vi "CLD 5 Parse Config Data File.vi"(8 "error in (no error)":errorcluster, 10 "Array In":T1[][](array[typedef])=[[{"Numeric"=1.25, "Boolean"=FALSE, "String"="One"}, {"Numeric"=1.35, "Boolean"=TRUE, "String"="Two"}, {"Numeric"=1.5, "Boolean"=FALSE, "String"="Three"}, {"Numeric"=1.0, "Boolean"=TRUE, "String"="Four"}], [{"Numeric"=2.0, "Boolean"=TRUE, "String"="Five"}, {"Numeric"=0.75, "Boolean"=FALSE, "String"="Six"}, {"Numeric"=0.9, "Boolean"=TRUE, "String"="Seven"}, {"Numeric"=0.75, "Boolean"=FALSE, "String"="Eight"}]], 11 "Get/Set":enum16{"Get", "Set"}(ring)) -> (0 "error out":errorcluster, 3 "Array Out":T1[][](array[typedef]))   [LabVIEW 2025]
doc: "CLD 5 exercise"
uses:
  CLD 5 Data Cluster.ctl
  <vilib>/Utility/config.llb/Read Key (Double).vi
  <vilib>/Utility/config.llb/Read Key (String).vi
  <vilib>/Utility/config.llb/Read Key (Boolean).vi
  <vilib>/Utility/config.llb/Read Key (I32).vi
  <vilib>/Utility/config.llb/Write Key (I32).vi
  <vilib>/Utility/config.llb/Write Key (String).vi
  <vilib>/Utility/config.llb/Write Key (Boolean).vi
  <vilib>/Utility/config.llb/Write Key (Double).vi
  <vilib>/Utility/config.llb/NI_LVConfig.lvlib
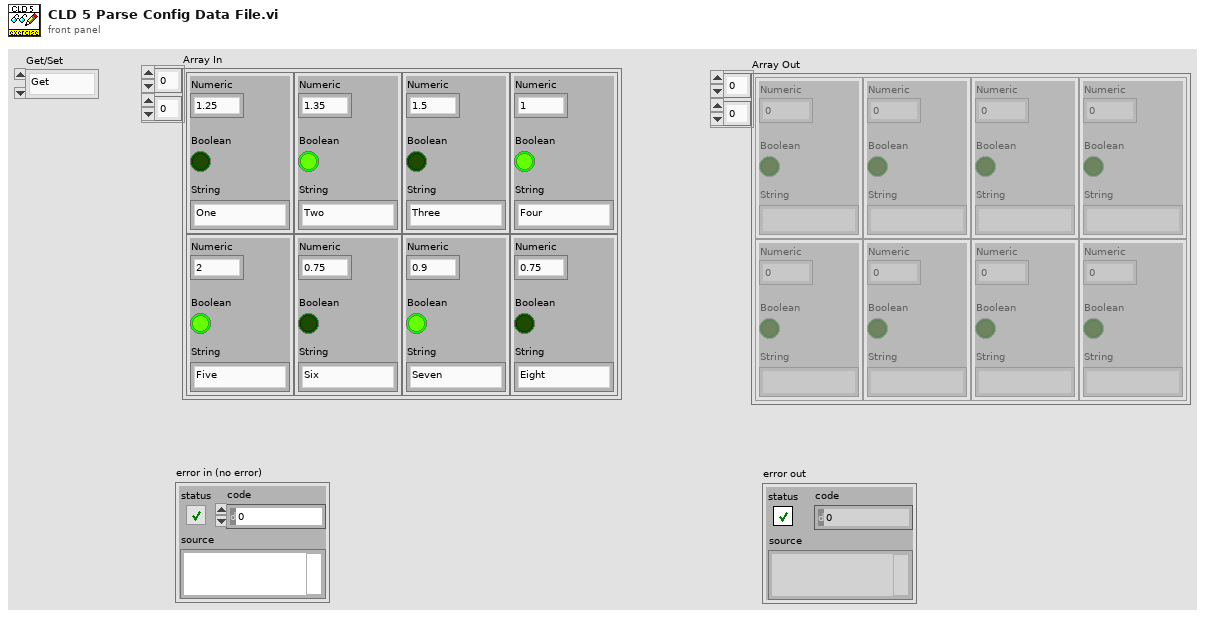
[diagram p1: front panel]
types:
  T1 = typedef "CLD 5 Data Cluster.ctl" = cluster{"Numeric":dbl, "Boolean":bool, "String":string}
  T2 = typedef "NI_LVConfig.lvlib/Config Data RefNum.ctl" = refnum<k1>
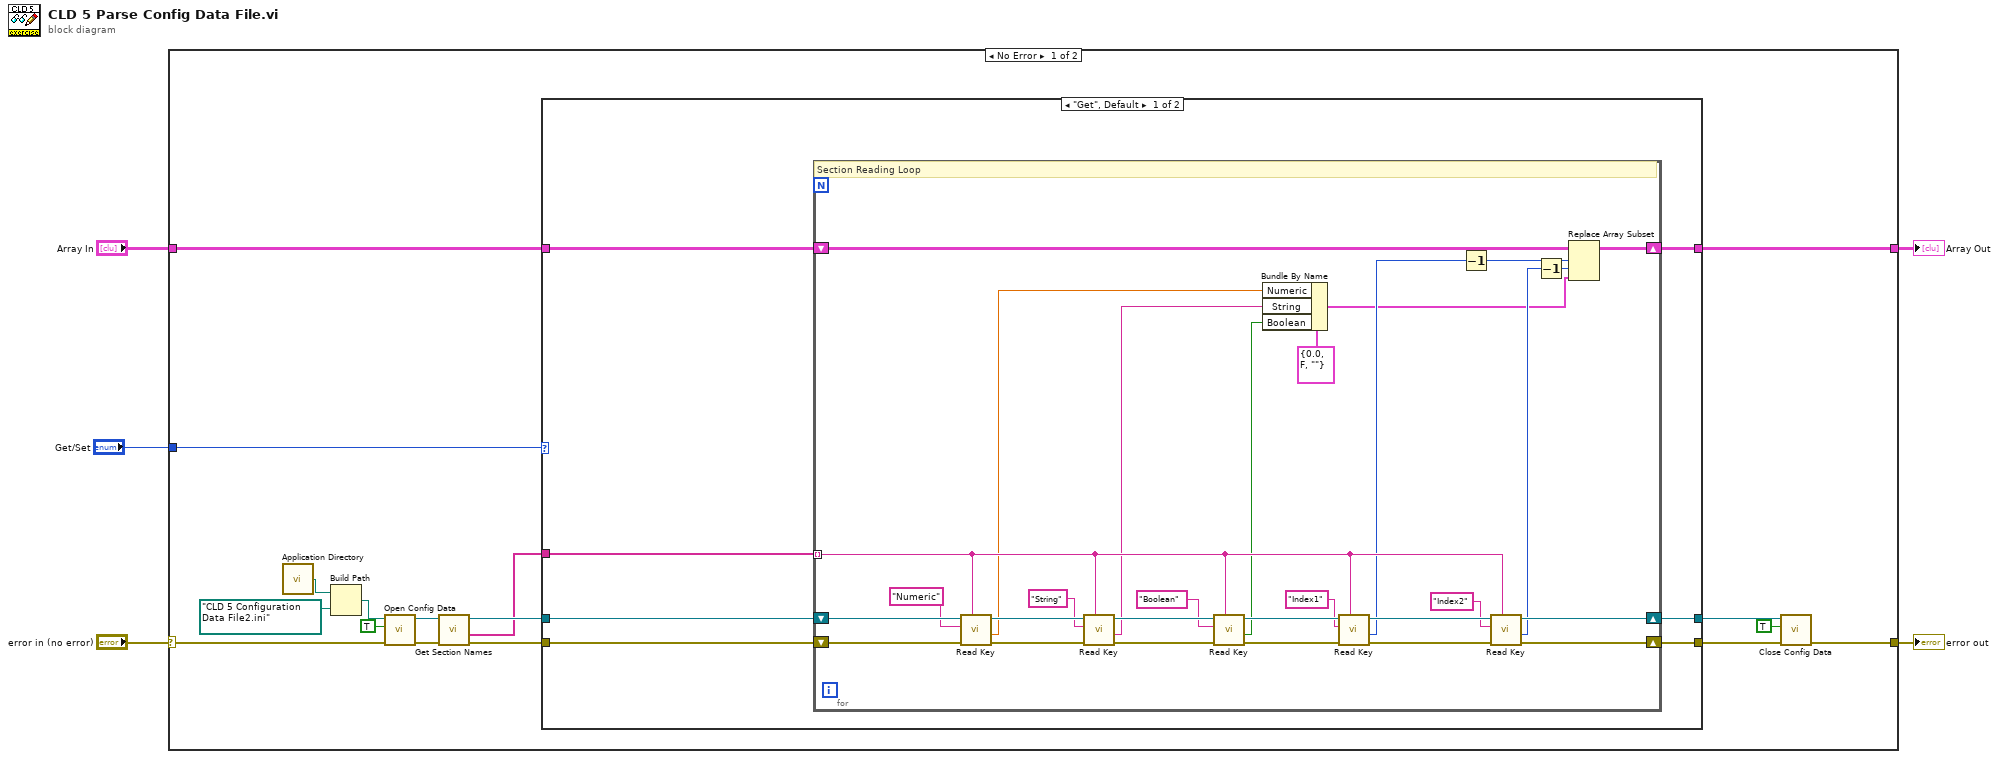
[diagram p0: block diagram]
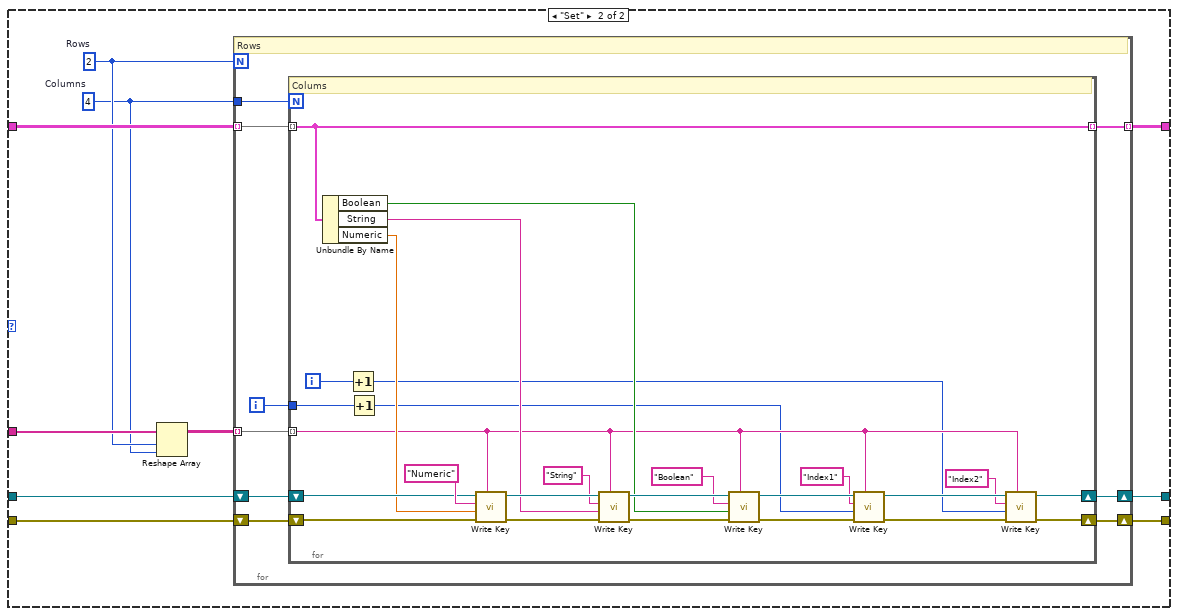
[diagram p2: hidden frame]
diagram:
  n1 = case shown="No Error" "error in (no error)" {
    selector: "error in (no error)" -> [w22 w105]
    tunnel: [w16 w105] -> w4
    tunnel: "Array In" -> [w20 w104]
    tunnel: [w19 w104] -> w2
    tunnel: "Get/Set" -> [w18 _]
    frame No Error {
      n2 = call <vilib>:"Application Directory.vi"() -> ("Application Directory"=w13:path)
      n3 = Build Path(base path=w13, name or relative path=path "CLD 5 Configuration Data File2.ini") -> (appended path=w14:path)
      n4 = call <vilib>:"Open Config Data.vi"("error in (no error)"=w22, "create file if necessary (T)"=TRUE, "configuration file path"=w14) -> ("error out"=w17:errorcluster, "refnum"=w9:T2)  [unwired: 6 in, 1 out]
      n5 = call <vilib>:"Get Section Names.vi"("error in (no error)"=w17, "refnum"=w9) -> ("error out"=w10:errorcluster, "section names"=w7:string[], "refnum out"=w8:T2)  [unwired: 7 in]
      n6 = case shown="\"Get\", Default" w18 {
        tunnel: w10 -> [w28 w68]
        tunnel: [w25 w65] -> w21
        tunnel: w20 -> [w29 w67]
        tunnel: [w26 w66] -> w19
        tunnel: w8 -> [w24 w64]
        tunnel: [w27 w63] -> w15
        tunnel: w7 -> [w23 w62]
        frame "Get", Default {
          n7 = for {
            shift-right: [w53] -> w25
            shift-left: w28 -> [w57]
            shift-right: [w55] -> w27
            shift-left: w24 -> [w56]
            tunnel: w23 -> [w44] mode=indexing
            shift-right: [w54] -> w26
            shift-left: w29 -> [w58]
            # "Section Reading Loop"
            n8 = call-poly <vilib>:"Read Key.vi"("section"=w44, "error in (no error)"=w57, "key"="Numeric", "refnum"=w56) -> ("error out"=w52:errorcluster, "value"=w37:dbl, "refnum out"=w50:T2)  [unwired: 4 in, 1 out]
            n9 = call-poly <vilib>:"Read Key.vi"("section"=w44, "error in (no error)"=w52, "key"="String", "refnum"=w50) -> ("error out"=w51:errorcluster, "value"=w36:string, "refnum out"=w48:T2)  [unwired: 4 in, 1 out]
            n10 = call-poly <vilib>:"Read Key.vi"("section"=w44, "error in (no error)"=w51, "key"="Boolean", "refnum"=w48) -> ("error out"=w49:errorcluster, "value"=w35:bool, "refnum out"=w46:T2)  [unwired: 4 in, 1 out]
            n11 = Bundle By Name(cluster=T1 {"Numeric"=0.0, "Boolean"=FALSE, "String"=""} ("Array"), "Numeric"=w37, "String"=w36, "Boolean"=w35) -> (w32:T1)
            n12 = call-poly <vilib>:"Read Key.vi"("section"=w44, "error in (no error)"=w49, "key"="Index1", "refnum"=w46) -> ("error out"=w47:errorcluster, "value"=w34:i32, "refnum out"=w45:T2)  [unwired: 4 in, 1 out]
            n13 = Decrement(x=w34) -> (x-1=w31:i32)
            n14 = call-poly <vilib>:"Read Key.vi"("section"=w44, "error in (no error)"=w47, "key"="Index2", "refnum"=w45) -> ("error out"=w53:errorcluster, "value"=w33:i32, "refnum out"=w55:T2)  [unwired: 4 in, 1 out]
            n15 = Decrement(x=w33) -> (x-1=w30:i32)
            n16 = Replace Array Subset(array=w58, new element=w32, index (row)=w31, index (col)=w30) -> (w54:T1[][])
          }
        }
        frame "Set" {
          w59 = 4  # Columns
          w60 = 2  # Rows
          n17 = Reshape Array "Reshape Array"(w62, w60, w59) -> (w61:string[][])
          n18 = for {
            N: w60 -> [_]
            tunnel: w67 -> [w76] mode=indexing
            tunnel: [w75] -> w66 mode=indexing
            shift-right: [w74] -> w65
            shift-left: w68 -> [w77]
            shift-right: [w72] -> w63
            shift-left: w64 -> [w73]
            tunnel: w61 -> [w70] mode=indexing
            tunnel: w59 -> [w69]
            i -> [w71]
            # "Rows"
            n19 = for {
              N: w69 -> [_]
              tunnel: w76 -> [w86] mode=indexing
              tunnel: [w86] -> w75 mode=indexing
              shift-right: [w87] -> w74
              shift-left: w77 -> [w90]
              shift-right: [w88] -> w72
              shift-left: w73 -> [w89]
              tunnel: w71 -> [w82]
              tunnel: w70 -> [w80] mode=indexing
              i -> [w81]
              # "Colums"
              n20 = Unbundle By Name(w86) -> ("Boolean"=w83:bool, "String"=w84:string, "Numeric"=w85:dbl)
              n21 = Increment(x=w81) -> (x+1=w79:i32)
              n22 = Increment(x=w82) -> (x+1=w78:i32)
              n23 = call-poly <vilib>:"Write Key.vi"("section"=w80, "error in (no error)"=w90, "value"=w85, "key"="Numeric", "refnum"=w89) -> ("error out"=w103:errorcluster, "refnum out"=w101:T2)  [unwired: 4 in, 1 out]
              n24 = call-poly <vilib>:"Write Key.vi"("section"=w80, "error in (no error)"=w103, "value"=w84, "key"="String", "refnum"=w101) -> ("error out"=w102:errorcluster, "refnum out"=w99:T2)  [unwired: 4 in, 1 out]
              n25 = call-poly <vilib>:"Write Key.vi"("section"=w80, "error in (no error)"=w102, "value"=w83, "key"="Boolean", "refnum"=w99) -> ("error out"=w100:errorcluster, "refnum out"=w97:T2)  [unwired: 4 in, 1 out]
              n26 = call-poly <vilib>:"Write Key.vi"("section"=w80, "error in (no error)"=w100, "value"=w78, "key"="Index1", "refnum"=w97) -> ("error out"=w98:errorcluster, "refnum out"=w96:T2)  [unwired: 4 in, 1 out]
              n27 = call-poly <vilib>:"Write Key.vi"("section"=w80, "error in (no error)"=w98, "value"=w79, "key"="Index2", "refnum"=w96) -> ("error out"=w87:errorcluster, "refnum out"=w88:T2)  [unwired: 4 in, 1 out]
            }
          }
        }
      }
      n28 = call <vilib>:"Close Config Data.vi"("error in (no error)"=w21, "write file if changed (T)"=TRUE, "refnum"=w15) -> ("error out"=w16:errorcluster)  [unwired: 7 in, 1 out]
    }
    frame Error {
    }
  }
  "error out" <- w4
  "Array Out" <- w2
